vi "CheckVersion.vi"(1 "Current Version":T1, 2 "New Version":T1) -> (0 "update":bool)   [LabVIEW 2014, in "Raspberry Pi Compatible Compiler for LabVIEW.lvlib" / "RasPiDownloader.lvlib"]
uses:
  RasPiDownloader.lvlib
  RuntimeVersion.ctl
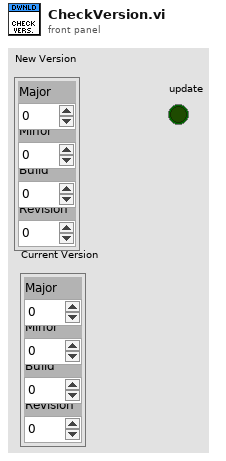
[diagram p1: front panel]
types:
  T1 = typedef "Raspberry Pi Compatible Compiler for LabVIEW.lvlib/RasPiDownloader.lvlib/RuntimeVersion.ctl" = cluster{"Major":i32, "Minor":i32, "Build":i32, "Revision":i32}
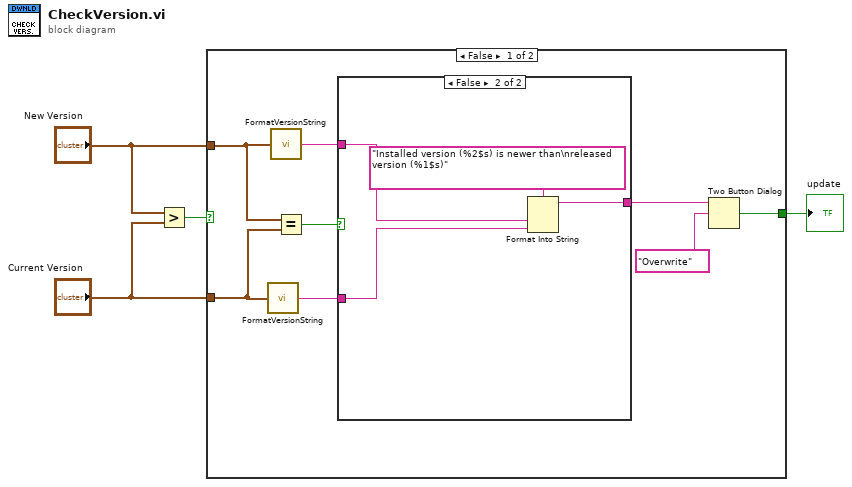
[diagram p0: block diagram]
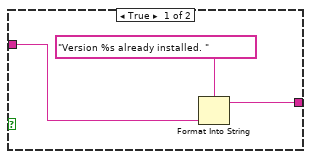
[diagram p2: hidden frame]
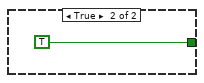
[diagram p3: hidden frame]
diagram:
  n1 = Greater?(x="New Version", y="Current Version") -> (0:w4:bool)
  n2 = case shown="False" w4 {
    tunnel: [w7 TRUE] -> w3
    tunnel: "New Version" -> [w12 _]
    tunnel: "Current Version" -> [w11 _]
    frame False {
      n3 = call "FormatVersionString.vi"("Version"=w11) -> ("Version string"=w8:string)  [unwired: 2 in]
      n4 = call "FormatVersionString.vi"("Version"=w12) -> ("Version string"=w9:string)  [unwired: 2 in]
      n5 = Equal?(x=w12, y=w11) -> (x = y?=w10:bool)
      n6 = case shown="False" w10 {
        tunnel: w9 -> [w15 w19]
        tunnel: w8 -> [_ w16]
        tunnel: [w14 w18] -> w6
        frame True {
          n7 = Format Into String(format string="Version %s already installed. ", w15) -> (resulting string=w14:string)  [unwired: 2 in, 1 out]
        }
        frame False {
          n8 = Format Into String(format string="Installed version (%2$s) is newer than\nreleased version (%1$s)", w19, w16) -> (resulting string=w18:string)  [unwired: 2 in, 1 out]
        }
      }
      n9 = Two Button Dialog(message=w6, 2:"Overwrite" ("T button name (\"OK\")")) -> (T button?=w7:bool)  [unwired: 1 in]
    }
    frame True {
    }
  }
  "update" <- w3
